vi "ICR_Reset_Hardware.vi"(8 "error in (no error)":errorcluster, 11 "QMH ICR Cluster":T2) -> (0 "error out":errorcluster, 3 "QMH ICR Cluster":T2)   [LabVIEW 2024]
doc: "This VI stops the hardware session of one sequence.\n\n1. Stop the waveform generation session for the HSDIO 6541 board.\n2. The other boards waiting for HSDIO should stop."
uses:
  controls/QMH_ICR_Cluster.ctl
  controls/HARDWARE_Resources.ctl
  controls/PROCESSING_Inputs.ctl
  controls/LOOPS_Inputs.ctl
  controls/OPO_Inputs.ctl
panel:
  in  "HARDWARE Resources":T1={"AO6711 Physical Channels"="Analog/ao0:3", "AO6711 Task Name"="", "AO_6738 Physical Channels"="AO_6738/ao0:3", "AO6738 Task Name"="", "AWG5421 Resource Name"="Waveform", "DIGIT 5122 Resource Name"="Digitizer", "HSDIO Resource Name"="Sequencer"}
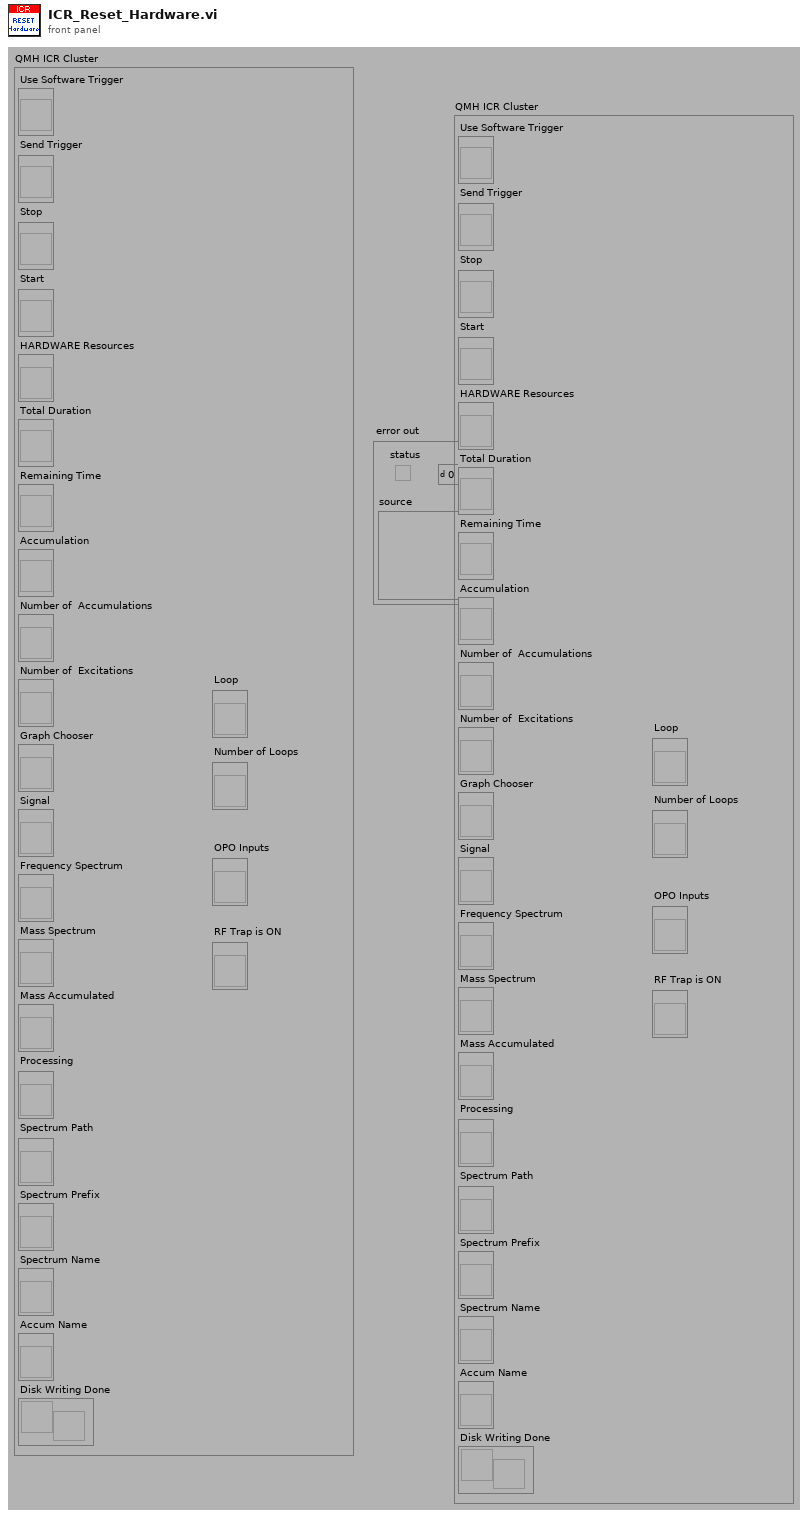
[diagram p1: front panel]
types:
  T1 = typedef "HARDWARE_Resources.ctl" = cluster{"AO6711 Physical Channels":tag, "AO6711 Task Name":refnum<k21>, "AO_6738 Physical Channels":tag, "AO6738 Task Name":refnum<k21>, "AWG5421 Resource Name":refnum<k15>, "DIGIT 5122 Resource Name":refnum<k15>, "HSDIO Resource Name":refnum<k15>}
  T2 = typedef "QMH_ICR_Cluster.ctl" = cluster{"Use Software Trigger":refnum<vi>, "Send Trigger":refnum<vi>, "Stop":refnum<vi>, "Start":refnum<vi>, "HARDWARE Resources":refnum<vi>, "Total Duration":refnum<vi>, "Remaining Time":refnum<vi>, "Accumulation":refnum<vi>, "Number of  Accumulations":refnum<vi>, "Number of  Excitations":refnum<vi>, "Graph Chooser":refnum<vi>, "Signal":refnum<vi>, "Frequency Spectrum":refnum<vi>, "Mass Spectrum":refnum<vi>, "Mass Accumulated":refnum<vi>, "Processing":refnum<vi>, "Spectrum Path":refnum<vi>, "Spectrum Prefix":refnum<vi>, "Spectrum Name":refnum<vi>, "Accum Name":refnum<vi>, "Disk Writing Done":refnum<notifier>, "Loop":refnum<vi>, "Number of Loops":refnum<vi>, "OPO Inputs":refnum<vi>, "RF Trap is ON":refnum<vi>}
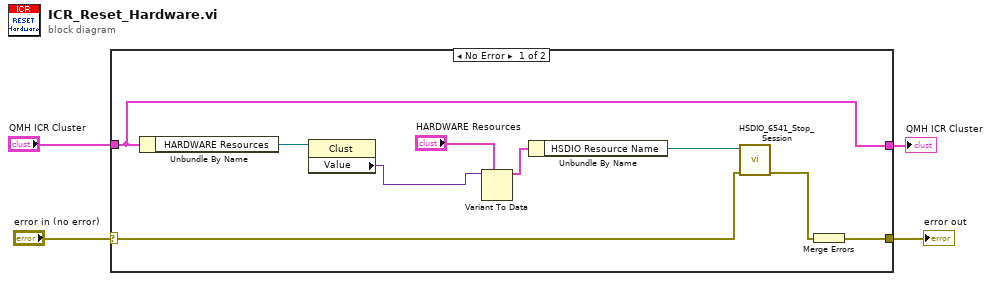
[diagram p0: block diagram]
diagram:
  n1 = case shown="No Error" "error in (no error)" {
    selector: "error in (no error)" -> [w5 w15]
    tunnel: [w11 w15] -> w4
    tunnel: "QMH ICR Cluster" -> [w6 w14]
    tunnel: [w6 w14] -> w1
    frame No Error {
      n2 = Unbundle By Name(w6) -> ("HARDWARE Resources"=w7:refnum<vi>)
      n3 = property class="Clust"(reference=w7) -> ("Value"=w10:variant)  [unwired: 1 in, 2 out]
      n4 = Variant To Data(type="HARDWARE Resources", Variant=w10) -> (data=w8:T1)  [unwired: 1 in, 1 out]
      n5 = Unbundle By Name(w8) -> ("HSDIO Resource Name"=w13:refnum<k15>)
      n6 = call "HSDIO_6541_Stop_Session.vi"("error in (no error)"=w5, "instrument handle in"=w13) -> ("error out"=w12:errorcluster)  [unwired: 9 in]
      n7 = Merge Errors(w12) -> (w11:errorcluster)
    }
    frame Error {
    }
  }
  "error out" <- w4
  "QMH ICR Cluster" <- w1
